vi "DashboardGetVariable.vi"(8 "Dashboard":refnum<k24>, 9 "name":string, 11 "error in":errorcluster) -> (0 "Response":cluster{"Message":string, "Succeed":bool}, 1 "Value":T1, 3 "error out":errorcluster)   [LabVIEW 2013, in "UnderAutomation.UniversalRobots.lvlib"]
uses:
  UnderAutomation.UniversalRobots.lvlib
  C:/Users/fg/Documents/UniversalRobots.vi/LabVIEW_2024/UnderAutomation.UniversalRobots/lib/UnderAutomation.UniversalRobots.dll
  LabVIEW_2024/UnderAutomation.UniversalRobots/lib/UnderAutomation.UniversalRobots.dll
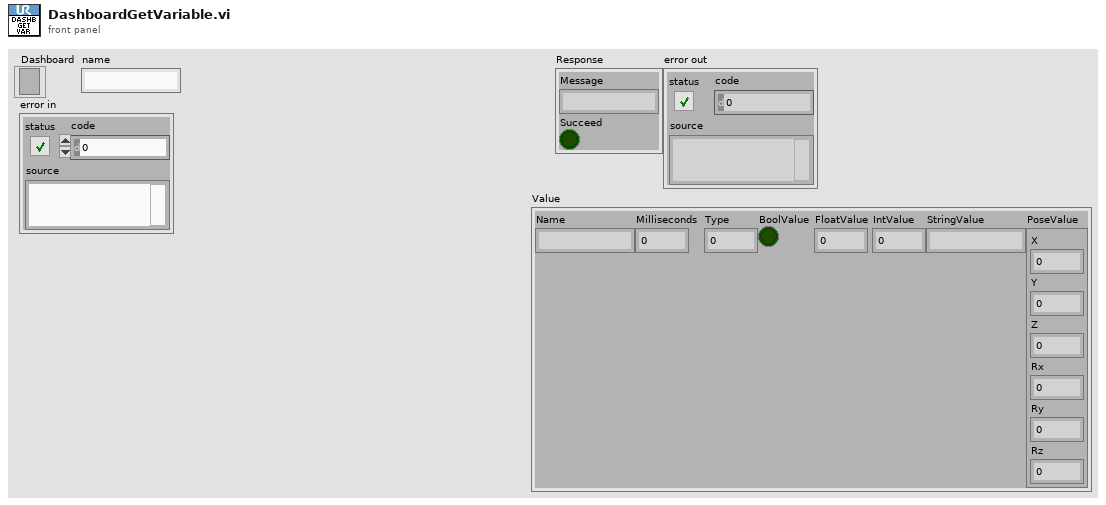
[diagram p1: front panel]
types:
  T1 = cluster{"Name":string, "Milliseconds":i32, "Type":i32, "BoolValue":bool, "FloatValue":sgl, "IntValue":i32, "StringValue":string, "PoseValue":cluster{"X":dbl, "Y":dbl, "Z":dbl, "Rx":dbl, "Ry":dbl, "Rz":dbl}}
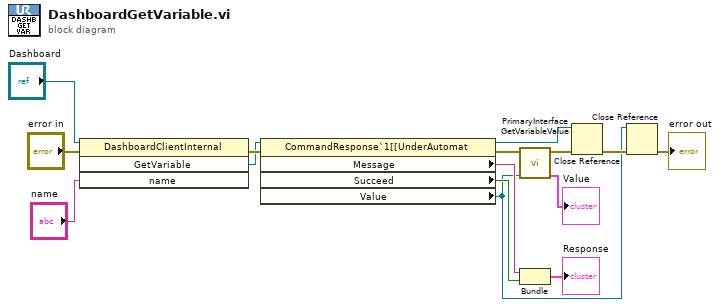
[diagram p0: block diagram]
diagram:
  n1 = invoke class="DashboardClientInternal" method="GetVariable"(reference="Dashboard", error in="error in", "name"="name") -> (error out=w10:errorcluster, "GetVariable"=w6:refnum<k24>)  [unwired: 1 in, 2 out]
  n2 = property class="CommandResponse`1[[UnderAutomat"(reference=w6, error in=w10) -> (reference out=w4:refnum<k24>, error out=w8:errorcluster, "Message"=w14:string, "Succeed"=w13:bool, "Value"=w1:refnum<k24>)
  n3 = call "PrimaryInterfaceGetVariableValue.vi"("Variable"=w1, "error in"=w8) -> ("Value"=→"Value":T1, "error out"=w5:errorcluster)  [unwired: 8 in]
  n4 = Bundle("Message"=w14, "Succeed"=w13) -> (→"Response":cluster{"Message":string, "Succeed":bool})  [unwired: 1 in]
  n5 = Close Reference(reference=w4, error in (no error)=w5) -> (error out=w3:errorcluster)
  n6 = Close Reference(reference=w1, error in (no error)=w3) -> (error out=→"error out":errorcluster)
